vi "Window-Speed graph length entry.vi"(8 "error in (no error)":errorcluster) -> (0 "error out (no error)":errorcluster, 3 "Cancelled":bool)   [LabVIEW 2013]
doc: "Use this template to create a dialog box with event handling."
uses:
  <vilib>/Utility/miscctls.llb/LVPointTypeDef.ctl
  Globals/gl_Time series viewer globals.vi
  Global Variables/General Globals.vi
panel:
  in  "Speed graph length":i32=10 min=1 max=60 format="%.0fs"
  in  "OK":bool
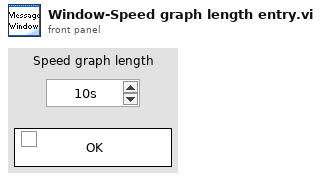
[diagram p1: front panel]
types:
  T1 = typedef "LVPointTypeDef.ctl" = cluster{"Horizontal":i16, "Vertical":i16}
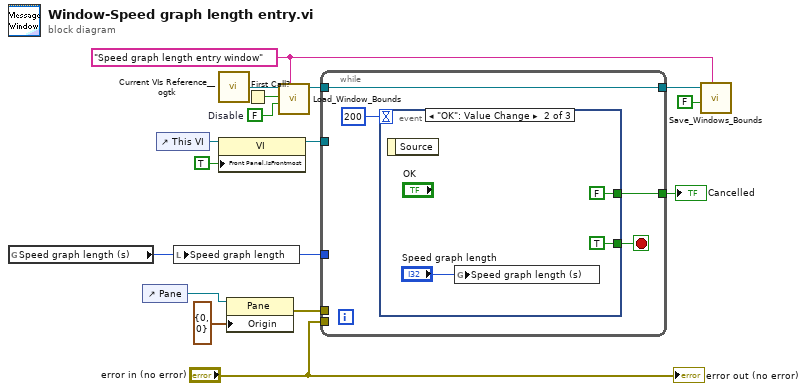
[diagram p0: block diagram]
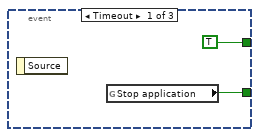
[diagram p2: hidden frame]
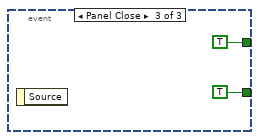
[diagram p3: hidden frame]
diagram:
  w8 = FALSE  # Disable
  w7 = "Speed graph length entry window" ("Window Name (i.e. Key)")
  n1 = global read "gl_Time series viewer globals.vi" "Speed graph length (s)"() -> (w2:i32)
  n2 = control-ref of="Pane"() -> (w11:refnum<vi>)
  n3 = control-ref of="This VI"() -> (w15:refnum<vi>)
  n4 = local write "Speed graph length"(w2) -> ()
  n5 = call "Current VIs Reference__ogtk.vi"() -> ("Current VI's reference"=w10:refnum<vi>)  [unwired: 5 in]
  n6 = property on="Property Node" class="VI"(reference=w15, "Front Panel.IsFrontmost"=TRUE ("Front Panel Window:Is Frontmost")) -> (reference out=w14:refnum<vi>)  [unwired: 1 in, 1 out]
  n7 = property class="Pane"(reference=w11, "Origin"=T1 {"Horizontal"=0, "Vertical"=0}) -> (error out=w12:errorcluster)  [unwired: 1 in, 1 out]
  n8 = First Call?() -> (First Call?: T/F=w9:bool)
  n9 = call "Load_Window_Bounds.vi"("Window Name (i.e. Key)"=w7, "Disable"=w8, "First Call"=w9, "Window VI's Ref"=w10) -> ("reference out"=w5:refnum<vi>)  [unwired: 4 in, 3 out]
  n10 = while {
    tunnel: w12 -> [_]
    tunnel: w14 -> [_]
    tunnel: w5 -> [w18]
    tunnel: [w18] -> w4
    tunnel: "error in (no error)" -> [_]
    tunnel: w2 -> [_]
    tunnel: [w17] -> w1
    stop <- w19 stop-if-true
    n11 = event shown="[1] \"OK\": Value Change" {
      selector: _ -> [_ _ _]
      dyn-events: _ -> [_ _ _]
      timeout: 200 -> [_ _ _]
      tunnel: [w22 TRUE ("Stop?") TRUE ("Stop?")] -> w19
      tunnel: [TRUE FALSE TRUE] -> w17
      event Timeout {
        n12 = event-data() -> ()  [unwired: 1 in, 1 out]
        n13 = global read "General Globals.vi" "Stop application"() -> (w22:bool)
      }
      event "OK": Value Change {
        n14 = event-data() -> ()  [unwired: 1 in, 1 out]
        n15 = global write "gl_Time series viewer globals.vi" "Speed graph length (s)"("Speed graph length") -> ()
      }
      event Panel Close {
        n16 = event-data() -> ()  [unwired: 1 in, 1 out]
      }
    }
  }
  "Cancelled" <- w1
  n17 = call "Save_Windows_Bounds.vi"("Window Name (i.e. Key)"=w7, "Front Panel Window:Open"=FALSE, "Window VI's Ref"=w4) -> ()  [unwired: 8 in, 1 out]
  "error out (no error)" <- "error in (no error)"
